vi "Uninit 1.vi"(2 "Container State":T1, 3 "Display State":T2) -> ()   [LabVIEW 2014, in "GCode_Xcontrol.xctl"]
uses:
  GCode_Xcontrol.xctl
  State 1.ctl
  <vilib>/_xctls/Container State.ctl
  <vilib>/_xctls/XControlSupport.lvlib
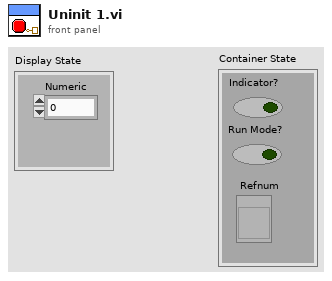
[diagram p1: front panel]
types:
  T1 = typedef "XControlSupport.lvlib/Container State.ctl" = cluster{"Indicator?":bool, "Run Mode?":bool, " Refnum":refnum<vi>}
  T2 = typedef "GCode_Xcontrol.xctl/State 1.ctl" = cluster{"Numeric":dbl}
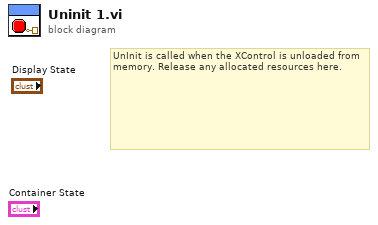
[diagram p0: block diagram]
diagram:
  # "UnInit is called when the XControl is unloaded from memory. Release any allocated resources here."
